vi "create data dictionary.vi"(8 "error in":errorcluster, 11 "system tags":refnum<class "data bus tag description.lvclass">[](array[class])) -> (0 "error out":errorcluster, 3 "data dictionary":refnum<class "data bus dictionary.lvclass">)   [LabVIEW 2013, in "data bus dictionary.lvclass"]
doc: "Accepts a set of tag descriptors and generates a fully formed data dictionary from these tags."
uses:
  data bus dictionary.lvclass
  tag/data bus tag description.lvclass
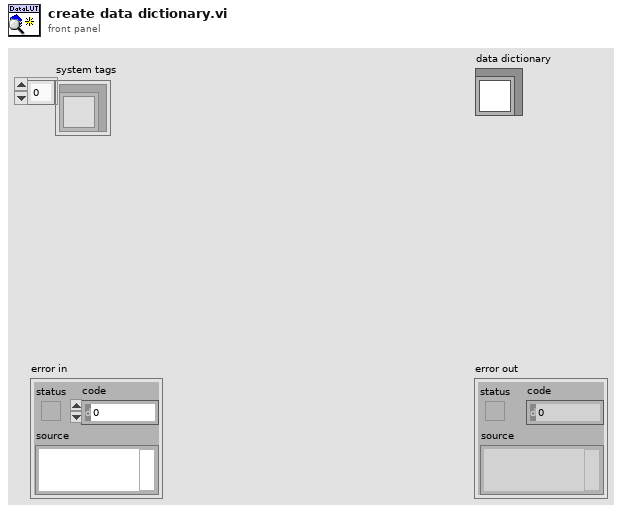
[diagram p1: front panel]
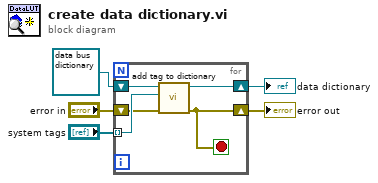
[diagram p0: block diagram]
diagram:
  n1 = for {
    shift-right: [w6] -> w1
    shift-left: "error in" -> [w8]
    shift-right: [w7] -> w2
    shift-left: refnum<class "data bus dictionary.lvclass"> refnum ("Data Locator in") -> [w10]
    tunnel: "system tags" -> [w9] mode=indexing
    stop <- w6 stop-if-true
    n2 = call "add tag to dictionary.vi"("error in"=w8, "system tag"=w9, "data dictionary in"=w10) -> ("error out"=w6:errorcluster, "data dictionary out"=w7:refnum<class "data bus dictionary.lvclass">)  [unwired: 7 in]
  }
  "error out" <- w1
  "data dictionary" <- w2
